vi "Get Motion Controller.vi"(8 "error in (no error)":errorcluster, 9 "Path":path, 10 "Section":string, 11 "Create Course Class in":refnum<class "Create Course Class.lvclass">) -> (0 "error out":errorcluster, 2 "iMotion Controller.lvclass":refnum<class "iMotion Controller.lvclass">, 3 "Create Course Class out":refnum<class "Create Course Class.lvclass">)   [LabVIEW 2022 SP3, in "Create Course Class.lvclass"]
uses:
  Create Course Class.lvclass
  Course SIM Motion Axis/Course SIM Motion Axis.lvclass
  iMotion Controller/iMotion Controller.lvclass
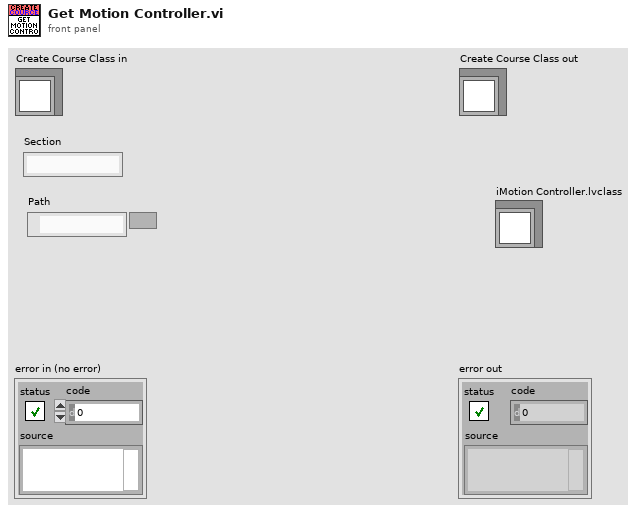
[diagram p1: front panel]
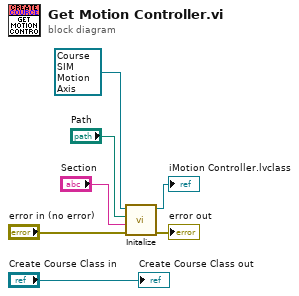
[diagram p0: block diagram]
diagram:
  n1 = call-dynamic "Initalize.vi"("error in (no error)"="error in (no error)", "Section"="Section", "Config Path"="Path", "Motion Controller in"=refnum<class "Course SIM Motion Axis.lvclass"> refnum ("Course SIM Motion Axis.lvclass")) -> ("error out"=→"error out":errorcluster, "Motion Controller out"=→"iMotion Controller.lvclass":refnum<class "Course SIM Motion Axis.lvclass">)  [unwired: 6 in]
  "Create Course Class out" <- "Create Course Class in"
